vi "crio_RT_Antagonist_New.vi"() -> ()   [LabVIEW 2019]
uses:
  <vilib>/Platform/TimedLoop/XDataNode/timing_clust.ctl
  <vilib>/Platform/TimedLoop/XDataNode/nitl_modes.ctl
  <vilib>/Platform/TimedLoop/XDataNode/wakeup.ctl
  <vilib>/FPGAPlugInAG/cRIO-9074/niLvFpga_Open_cRIO-9074.vi
  <vilib>/rvi/interface/common/dynamic/niFpgaDynamicAddResources.vi
  <vilib>/Utility/error.llb/Error Cluster From Error Code.vi
  <vilib>/rvi/errors/niLvFpgaAdjustHostInterfaceError.vi
  <vilib>/FPGAPlugInAG/Dynamic/niLvFpga_Close_Dynamic.vi
  <vilib>/rvi/interface/nirviOpenFPGA/nirviOpenFPGA.xnode
  FPGA Bitfiles/gpass2_FPGATarget2_crioFPGAAntagoni_cDOKBUczdNQ.lvbitx
  crio_FPGA_Antagonist_Radial.vi
  <vilib>/rvi/interface/nirviReadWriteControl/nirviReadWriteControl.xnode
  <vilib>/platform/TimedLoop/XDataNode/XDataNode.xnode
  <vilib>/rvi/interface/nirviCloseFPGA/nirviCloseFPGA.xnode
  NiFpgaLv.dll
  <vilib>/rvi/interface/Simulation/niFpgaSimulationCallBeginRW.vi
  <vilib>/Platform/TimedLoop/XDataNode/XDNodeRunTimeDep.lvlib
panel:
  out "Rail Position":i16(graph)
  out "rail Platform Position":i16
  in  "Half Peirod (pulse 40MHz)":u32=10000
  in  "Rail Desired Position":i16(slide) scale=0.0..20000.0
  in  "Rail Stepper Direction":bool
  in  "Rail Stepper Enable":bool
  in  "Rail Manual Operation":bool
  in  "Autolock":bool
  out "LAC Measured Position":i32(graph)
  out "LAC Measured Position":i32
  in  "LAC manual control":T1={"manual? (F)"=FALSE, "manual input (0)"=-0.83838385} {"manual input (0)" scale=-1.0..1.0}
  in  "LAC Position Reset":bool
  in  "LAC Gains":T2={"proportional gain"=0.95454544, "integral gain"=0.64646465} {"proportional gain" scale=0.0..1.0; "integral gain" scale=0.0..1.0}
  in  "LAC Velocity Interval (uSec)":u32=1000
  in  "LAC setpoint":i32(slide) scale=0.0..4500.0
  out "LAC Actual Gain":T2={"proportional gain"=0.009545455, "integral gain"=1.2626262e-09}
  in  "LAC Gain Scaler":T2={"proportional gain"=100.0, "integral gain"=100000000.0}
  in  "stop":bool
  out "VCA Measured Velocity (Counts/Interval)":i32
  out "VCA Controller PWM Output":sgl=-0.35149753
  out "VCA Measured Position":i32=4
  in  "VCA Loop Period(us)":i64=2000
  out "VCA Measured Position":i32(graph)=4
  in  "VCA  manual control":T1 {"manual input (0)" scale=-1.0..1.0}
  in  "VCA Position Reset":bool
  in  "VCA Gains":T2={"proportional gain"=0.97979796, "integral gain"=0.7979798} {"proportional gain" scale=0.0..1.0; "integral gain" scale=0.0..1.0}
  in  "VCA Velocity Interval (uSec)":u32=1000
  in  "VCA setpoint":i32(slide) scale=0.0..2700.0
  out "VCA Actual Gain":T2={"proportional gain"=0.0009797979, "integral gain"=7.979798e-09}
  in  "VCA Gain Scaler":T2={"proportional gain"=1000.0, "integral gain"=100000000.0}
  in  "PWM Frequency (default 20kHz)":i32=20000
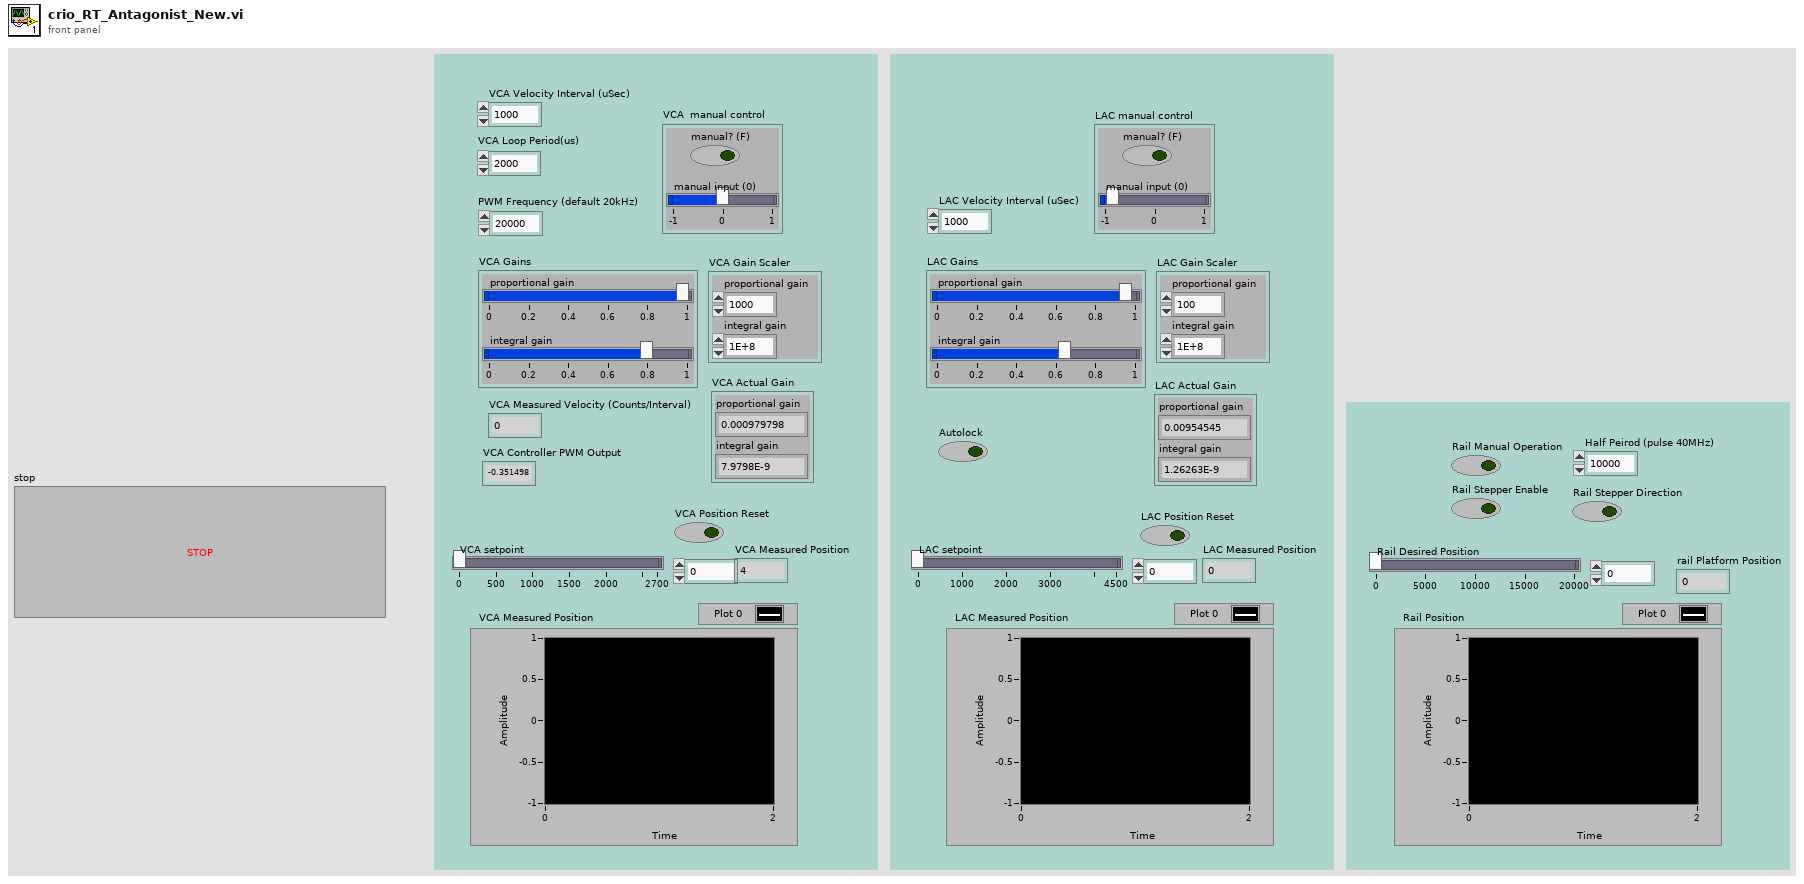
[diagram p1: front panel]
types:
  T1 = cluster{"manual? (F)":bool, "manual input (0)":sgl}
  T2 = cluster{"proportional gain":sgl, "integral gain":sgl}
  T3 = typedef "XDNodeRunTimeDep.lvlib/timing_clust.ctl" = cluster{"Expected End [f-1]":u64, "Actual End [f-1]":u64, "Finished Late? [f-1]":bool, "Expected End [i-1]":u64, "Actual End [i-1]":u64, "Finished Late? [i-1]":bool, "Expected Start [i]":u64, "Actual Start [i]":u64, "Expected Start [f]":u64, "Actual Start [f]":u64, "Source Name":string, "Structure Name":string, "Period":i64, "Deadline":i64, "Offset":i64, "Start":i64, "Priority":i32, "Timeout":i32, "Mode":T4, "Wakeup Reason":T5, "Error":errorcluster, "Source Type":string, "Secondary Source Type":string, "Global End Time":u64, "Global Start Time":u64, "Frame Duration":u64, "Iteration Duration":u64, "Assigned CPU":i32, "I/O Scan Engine Mode":u32}
  T4 = typedef "XDNodeRunTimeDep.lvlib/nitl_modes.ctl" = enum32{"No Change", "Process missed periods, maintain original phase", "Discard missed periods, maintain original phase", "Process missed periods, ignore original phase", "Discard missed periods, ignore original phase"}
  T5 = typedef "XDNodeRunTimeDep.lvlib/wakeup.ctl" = enum32{"Normal", "Aborted", "Asynchronous wakeup", "Timing source error", "Timed loop error", "Timeout"}
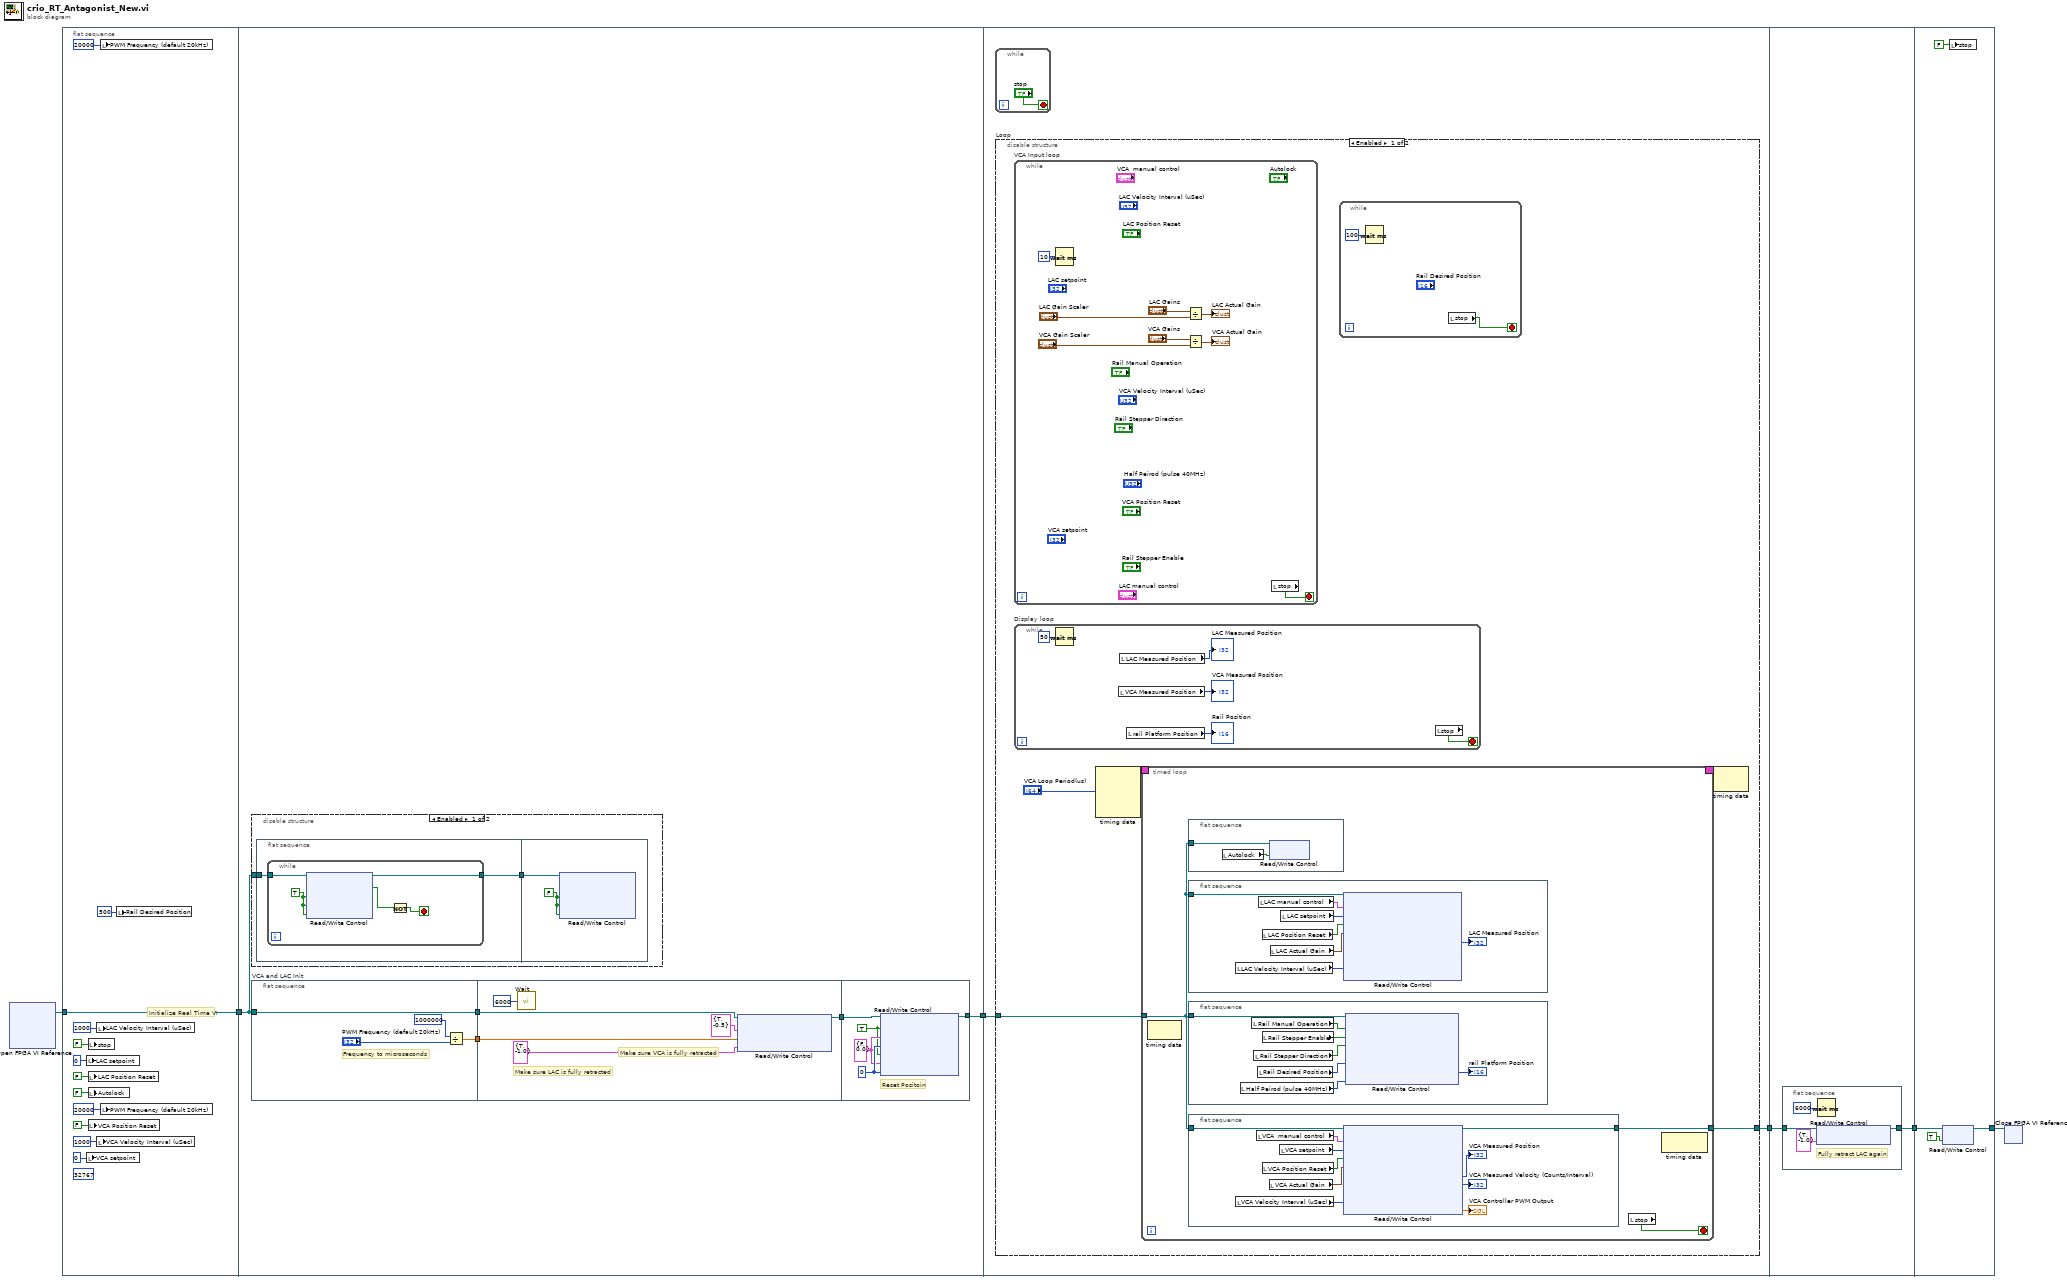
[diagram p0: block diagram]
diagram:
  n1 = xnode "Open FPGA VI Reference"() -> ("FPGA VI Reference Out"=w6:refnum<k20>)  [unwired: 2 in, 1 out]
  n2 = flat-sequence {
    tunnel: w6 -> [w17]
    tunnel: [w17] -> w5
    tunnel: [w23] -> w4
    tunnel: w5 -> [w19]
    tunnel: w4 -> [w51]
    tunnel: [w50] -> w2
    tunnel: w2 -> [w109]
    tunnel: [w108] -> w1
    tunnel: w1 -> [w117]
    tunnel: [w116] -> w3
    frame #0 {
      (unwired) i16 32767 ("Initialize Rail Position")
      # "Initialize Real Time VI"
      n3 = local write "LAC setpoint"(0 ("VCA setpoint")) -> ()
      n4 = local write "VCA setpoint"(0 ("VCA setpoint")) -> ()
      n5 = local write "stop"(FALSE ("stop")) -> ()
      n6 = local write "LAC Position Reset"(FALSE ("VCA Position Reset")) -> ()
      n7 = local write "Autolock"(FALSE ("Autolock")) -> ()
      n8 = local write "VCA Position Reset"(FALSE ("VCA Position Reset")) -> ()
      n9 = local write "LAC Velocity Interval (uSec)"(u32 1000 ("Velocity Interval (uSec)")) -> ()
      n10 = local write "VCA Velocity Interval (uSec)"(u32 1000 ("Velocity Interval (uSec)")) -> ()
      n11 = local write "PWM Frequency (default 20kHz)"(20000 ("PWM Frequency")) -> ()
      n12 = local write "PWM Frequency (default 20kHz)"(20000 ("PWM Frequency (default 20kHz)")) -> ()
      n13 = local write "Rail Desired Position"(i16 500 ("Rail Desired Position")) -> ()
    }
    frame #1 {
      n14 = disable-structure shown="Enabled" {
        disable-tunnel: w19 -> [w24 _]
        frame Enabled {
          n15 = flat-sequence {
            tunnel: w24 -> [w26]
            tunnel: [w27] -> w25
            tunnel: w25 -> [w34]
            frame #0 {
              n16 = while {
                tunnel: [w31] -> w27
                tunnel: w26 -> [w30]
                stop <- w28 stop-if-true
                w32 = TRUE ("Stepper Direction")
                n17 = xnode "Read/Write Control"("FPGA VI Reference In"=w30, "Manual Operation"=w32, "Stepper Enable"=w32, "Stepper Direction"=w32) -> ("FPGA VI Reference Out"=w31:refnum<k20>, "Limit Switch"=w29:bool)  [unwired: 1 in, 1 out]
                n18 = Not(x=w29) -> (.not. x?=w28:bool)
              }
            }
            frame #1 {
              w33 = FALSE ("Stepper Direction")
              n19 = xnode "Read/Write Control"("FPGA VI Reference In"=w34, "Manual Operation"=w33, "Stepper Enable"=w33, "Stepper Direction"=w33) -> ()  [unwired: 1 in, 3 out]
            }
          }
        }
        frame Disabled {
        }
      }
      n20 = flat-sequence "VCA and LAC Init" {
        tunnel: [w37] -> w22
        tunnel: w19 -> [w35]
        tunnel: [w35] -> w21
        tunnel: w22 -> [w43]
        tunnel: w21 -> [w39]
        tunnel: [w44] -> w20
        tunnel: w20 -> [w48]
        tunnel: [w49] -> w23
        frame #0 {
          # "Frequency to microseconds"
          n21 = Divide(x=1000000, y="PWM Frequency (default 20kHz)") -> (x/y=w37:dbl)
        }
        frame #1 {
          # "Make sure LAC is fully retracted"
          # "Make sure VCA is fully retracted"
          n22 = call "Wait"("Count(mSec)"=u32 6000) -> ()  [unwired: 1 out]
          n23 = xnode "Read/Write Control"("FPGA VI Reference In"=w39, "VCA Manual Control"=T1 {"manual? (F)"=TRUE, "manual input (0)"=-0.5} ("manual control"), "DC PWM Period (microsec)"=w43, "LAC Manual Control"=T1 {"manual? (F)"=TRUE, "manual input (0)"=-1.0} ("manual control")) -> ("FPGA VI Reference Out"=w44:refnum<k20>)  [unwired: 1 in, 1 out]
        }
        frame #2 {
          w47 = 0 ("setpoint")
          w46 = T1 {"manual? (F)"=FALSE, "manual input (0)"=0.0} ("manual control")
          w45 = TRUE ("Position Reset")
          # "Reset Positoin"
          n24 = xnode "Read/Write Control"("FPGA VI Reference In"=w48, "VCA Position Reset"=w45, "VCA Manual Control"=w46, "VCA Position Setpoint"=w47, "Position Reset"=w45, "LAC Manual Control"=w46, "LAC Setpoint"=w47) -> ("FPGA VI Reference Out"=w49:refnum<k20>)  [unwired: 1 in, 1 out]
        }
      }
    }
    frame #2 {
      n25 = while {
        stop <- "stop" stop-if-true
      }
      n26 = disable-structure "Loop" shown="Enabled" {
        disable-tunnel: w51 -> [w53 _]
        disable-tunnel: [w52 _] -> w50
        frame Enabled {
          n27 = while "VCA Input loop" {
            stop <- w65 stop-if-true
            n28 = Wait (ms)(milliseconds to wait=u32 10) -> ()  [unwired: 1 out]
            n29 = Divide(x="LAC Gains", y="LAC Gain Scaler") -> (x/y=→"LAC Actual Gain":T2)
            n30 = Divide(x="VCA Gains", y="VCA Gain Scaler") -> (x/y=→"VCA Actual Gain":T2)
            n31 = local read "stop"() -> (w65:bool)
          }
          n32 = while "Display loop" {
            stop <- w70 stop-if-true
            n33 = Wait (ms)(milliseconds to wait=u32 50) -> ()  [unwired: 1 out]
            n34 = local read "VCA Measured Position"() -> (→"VCA Measured Position":i32)
            n35 = local read "LAC Measured Position"() -> (→"LAC Measured Position":i32)
            n36 = local read "rail Platform Position"() -> (→"Rail Position":i16)
            n37 = local read "stop"() -> (w70:bool)
          }
          n38 = node-c288("VCA Loop Period(us)") -> (w56:T3)  [unwired: 3 in]
          n39 = timed-loop {
            timing: w56 -> [_]
            timing-out: [_] -> w55
            tunnel: w53 -> [w72]
            tunnel: [w74] -> w52
            stop <- w73 stop-if-true
            n40 = node-c288() -> ()  [unwired: 1 in, 1 out]
            n41 = flat-sequence {
              tunnel: w72 -> [w83]
              frame #0 {
                n42 = local read "Autolock"() -> (w82:bool)
                n43 = xnode "Read/Write Control"("FPGA VI Reference In"=w83, "LAC Lock"=w82) -> ()  [unwired: 1 in, 2 out]
              }
            }
            n44 = flat-sequence {
              tunnel: w72 -> [w90]
              frame #0 {
                n45 = local read "LAC Velocity Interval (uSec)"() -> (w85:u32)
                n46 = local read "LAC manual control"() -> (w89:T1)
                n47 = local read "LAC Position Reset"() -> (w87:bool)
                n48 = local read "LAC Actual Gain"() -> (w86:T2)
                n49 = local read "LAC setpoint"() -> (w88:i32)
                n50 = xnode "Read/Write Control"("FPGA VI Reference In"=w90, "LAC Manual Control"=w89, "LAC Setpoint"=w88, "Position Reset"=w87, "LAC Gains"=w86, "LAC Velocity Interval (uSec)"=w85) -> ("LAC Position (Counts)"=→"LAC Measured Position":i32)  [unwired: 1 in, 5 out]
              }
            }
            n51 = flat-sequence {
              tunnel: w72 -> [w75]
              frame #0 {
                n52 = local read "Half Peirod (pulse 40MHz)"() -> (w81:u32)
                n53 = local read "Rail Manual Operation"() -> (w77:bool)
                n54 = local read "Rail Stepper Direction"() -> (w78:bool)
                n55 = local read "Rail Desired Position"() -> (w80:i16)
                n56 = local read "Rail Stepper Enable"() -> (w79:bool)
                n57 = xnode "Read/Write Control"("FPGA VI Reference In"=w75, "Manual Operation"=w77, "Stepper Enable"=w79, "Stepper Direction"=w78, "Position Control: Desired Positoin"=w80, "Half Peirod (pulse 40MHz)"=w81) -> ("rail Platform Position"=→"rail Platform Position":i16)  [unwired: 2 in, 2 out]
              }
            }
            n58 = flat-sequence {
              tunnel: [w93] -> w74
              tunnel: w72 -> [w92]
              frame #0 {
                n59 = local read "VCA Velocity Interval (uSec)"() -> (w91:u32)
                n60 = local read "VCA  manual control"() -> (w94:T1)
                n61 = local read "VCA Position Reset"() -> (w97:bool)
                n62 = local read "VCA Actual Gain"() -> (w96:T2)
                n63 = local read "VCA setpoint"() -> (w95:i32)
                n64 = xnode "Read/Write Control"("FPGA VI Reference In"=w92, "VCA Manual Control"=w94, "VCA Position Setpoint"=w95, "VCA Position Reset"=w97, "VCA Gains"=w96, "Velocity Interval (uSec)"=w91) -> ("FPGA VI Reference Out"=w93:refnum<k20>, "Position (Counts) VCA"=→"VCA Measured Position":i32, "Velocity (Counts/Interval) VCA"=→"VCA Measured Velocity (Counts/Interval)":i32, "VCA ControllerPWM Output"=→"VCA Controller PWM Output":sgl)  [unwired: 1 in, 2 out]
              }
            }
            n65 = local read "stop"() -> (w73:bool)
            n66 = node-c288() -> ()  [unwired: 1 in, 1 out]
          }
          n67 = while {
            stop <- w57 stop-if-true
            n68 = Wait (ms)(milliseconds to wait=u32 100) -> ()  [unwired: 1 out]
            n69 = local read "stop"() -> (w57:bool)
          }
          n70 = node-c288(w55) -> ()  [unwired: 1 out]
        }
        frame Disabled {
        }
      }
    }
    frame #3 {
      n71 = flat-sequence {
        tunnel: w109 -> [w112]
        tunnel: [w111] -> w108
        frame #0 {
          # "Fully retract LAC again"
          n72 = xnode "Read/Write Control"("FPGA VI Reference In"=w112, "LAC Manual Control"=T1 {"manual? (F)"=TRUE, "manual input (0)"=-1.0}) -> ("FPGA VI Reference Out"=w111:refnum<k20>)  [unwired: 1 in, 1 out]
          n73 = Wait (ms)(milliseconds to wait=u32 6000) -> ()  [unwired: 1 out]
        }
      }
    }
    frame #4 {
      n74 = xnode "Read/Write Control"("FPGA VI Reference In"=w117, "stop"=TRUE) -> ("FPGA VI Reference Out"=w116:refnum<k20>)  [unwired: 1 in, 1 out]
      n75 = local write "stop"(FALSE ("stop")) -> ()
    }
  }
  n76 = xnode "Close FPGA VI Reference"("FPGA VI Reference In"=w3) -> ()  [unwired: 1 in, 1 out]
